vi "Preselection_KBC22_32.vi"(0 "SI804.lvclass":refnum<class "SI804.lvclass">, 5 "3 JSC30 DG801\nXA12":bool, 7 "3 JSC30 DG802\nXA12":bool, 11 "error in":errorcluster) -> (4 "SI804.lvclass out":refnum<class "SI804.lvclass">, 6 "PreSelec KBC22":bool, 8 "PreSelec KBC32":bool, 15 "error out":errorcluster)   [LabVIEW 2022 SP3, in "SI804.lvclass"]
uses:
  SI804.lvclass
  SI804.lvclass/SI804.ctl
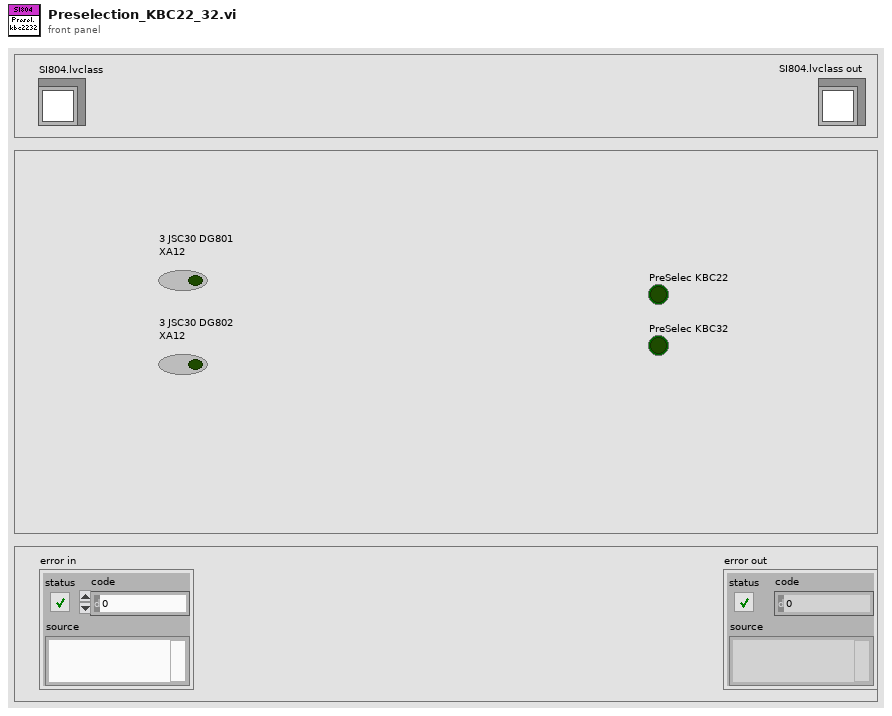
[diagram p1: front panel]
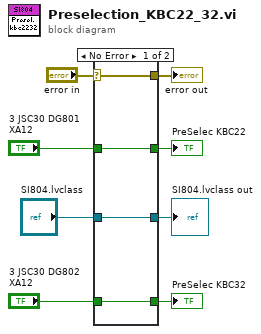
[diagram p0: block diagram]
diagram:
  n1 = case shown="No Error" "error in" {
    selector: "error in" -> [w10 w13]
    tunnel: "3 JSC30 DG801\nXA12" -> [w12 _]
    tunnel: "3 JSC30 DG802\nXA12" -> [w11 _]
    tunnel: [w12 _] -> w5
    tunnel: [w11 _] -> w4
    tunnel: [w10 w13] -> w3
    tunnel: "SI804.lvclass" -> [w9 w14]
    tunnel: [w9 w14] -> w1
    frame No Error {
    }
    frame Error {
    }
  }
  "PreSelec KBC22" <- w5
  "PreSelec KBC32" <- w4
  "error out" <- w3
  "SI804.lvclass out" <- w1
